vi "IsConnected.vi"(8 "error in (no error)":errorcluster, 11 "NetworkStreamReader in":refnum<class "NetworkStreamReader.lvclass">) -> (0 "error out":errorcluster, 2 "Connected?":bool, 3 "NetworkStreamReader out":refnum<class "NetworkStreamReader.lvclass">)   [LabVIEW 2011, in "NetworkStreamReader.lvclass"]
uses:
  NetworkStreamReader.lvclass
  NetworkStreamReader.lvclass/NetworkStreamReader.ctl
  Program Files/National Instruments/LabVIEW 2011/resource/objmgr/ni.dex.rc
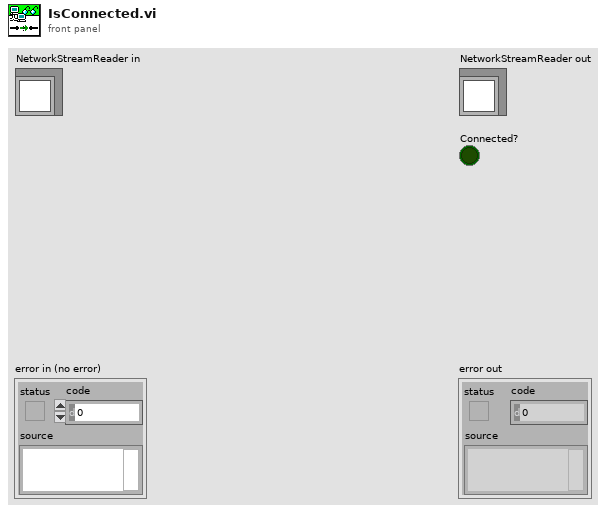
[diagram p1: front panel]
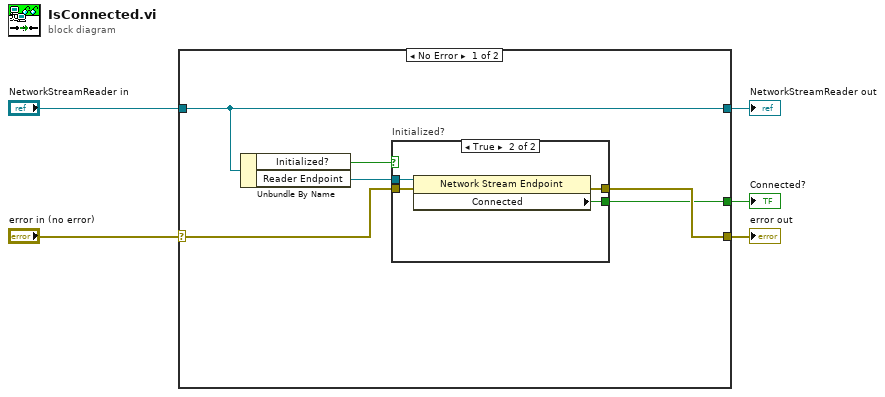
[diagram p0: block diagram]
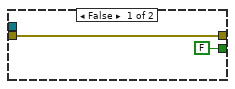
[diagram p2: hidden frame]
diagram:
  n1 = case shown="No Error" "error in (no error)" {
    selector: "error in (no error)" -> [w8 w19]
    tunnel: [w7 w19] -> w4
    tunnel: [w11 w18] -> w2
    tunnel: "NetworkStreamReader in" -> [w11 w18]
    tunnel: [w6 _] -> w1
    frame No Error {
      n2 = Unbundle By Name(w11) -> ("Initialized?"=w10:bool, "Reader Endpoint"=w9:refnum<k21>)
      n3 = case "Initialized?" shown="True" w10 {
        tunnel: w9 -> [_ w17]
        tunnel: w8 -> [w12 w16]
        tunnel: [w12 w15] -> w7
        tunnel: [FALSE ("Connected") w14] -> w6
        frame False {
        }
        frame True {
          n4 = property class="Network Stream Endpoint"(reference=w17, error in=w16) -> (error out=w15:errorcluster, "Connected"=w14:bool)  [unwired: 1 out]
        }
      }
    }
    frame Error {
    }
  }
  "error out" <- w4
  "NetworkStreamReader out" <- w2
  "Connected?" <- w1
